vi "stupid put action.vi"(7 "transmit queue":refnum<queue>, 11 "application request in":T1) -> (0 "connection error":errorcluster)   [LabVIEW 2016]
uses:
  HTTP server/http request.ctl
  HTTP server/http method.ctl
  HTTP headers/http header data.ctl
  HTTP server/http response.ctl
  HTTP server/http response packet type.ctl
  HTTP headers/http add header to set.vi
  HTTP server/Basic HTTP server.lvclass
  HTTP headers/http headers.lvlib
  HTTP responder/http responder.lvclass
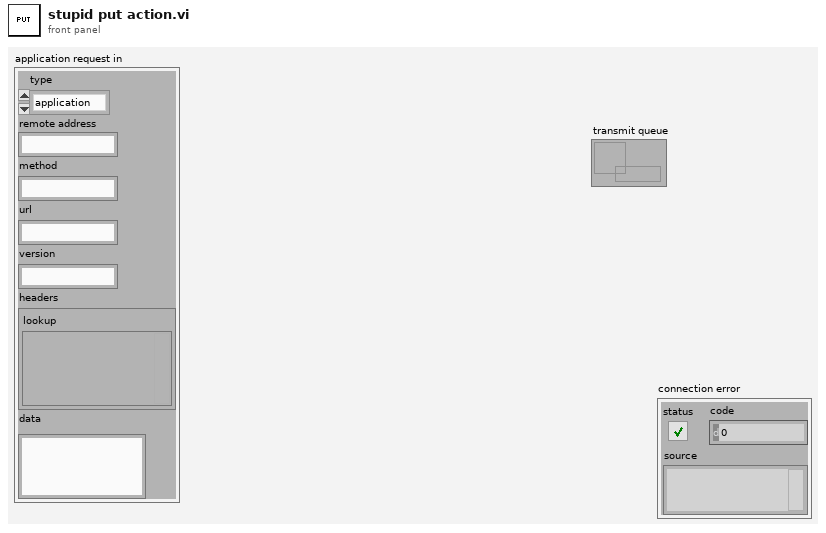
[diagram p1: front panel]
types:
  T1 = typedef "Basic HTTP server.lvclass/http request.ctl" = cluster{"type":T2, "remote address":string, "method":string, "url":string, "version":string, "headers":T3, "data":string}
  T2 = typedef "Basic HTTP server.lvclass/http method.ctl" = enum16{"application", "error", "upgrade", "expect"}
  T3 = typedef "http headers.lvlib/http header data.ctl" = cluster{"lookup":variant}
  T4 = typedef "Basic HTTP server.lvclass/http response packet type.ctl" = enum16{"full response", "header only", "data only", "last data", "raw output"}
  T5 = typedef "Basic HTTP server.lvclass/http response.ctl" = cluster{"packet type":T4, "reason code":u16, "status string":string, "headers":T3, "cookies":string[], "data":string}
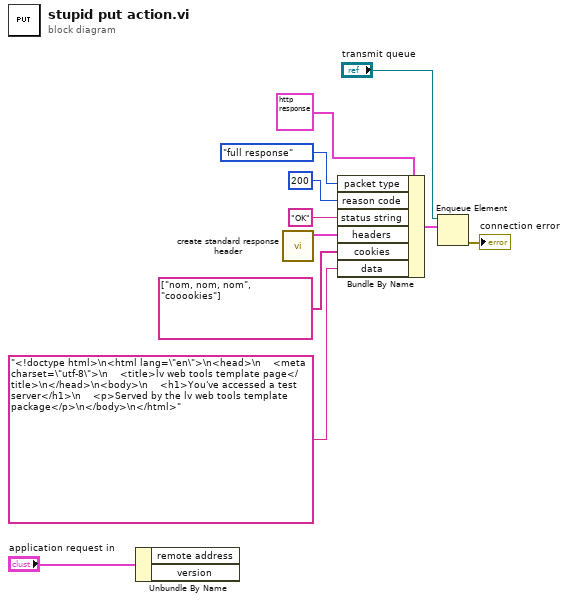
[diagram p0: block diagram]
diagram:
  n1 = Unbundle By Name("application request in") -> ()  [unwired: 2 out]
  n2 = call "create standard response header.vi"() -> ("default header"=w2:T3)  [unwired: 11 in]
  n3 = Bundle By Name(cluster=T5 {"packet type"=enum."full response", "reason code"=0, "status string"="", "headers"={"lookup"=variant}, "cookies"=[], "data"=""} ("application request"), "packet type"=http_response_packet_type."full response", "reason code"=u16 200, "status string"="OK", "headers"=w2, "cookies"=string[] ["nom, nom, nom", "cooookies"], "data"="<!doctype html>\n<html lang=\"en\">\n<head>\n    <meta charset=\"utf-8\">\n    <title>lv web tools template page</title>\n</head>\n<body>\n    <h1>You've accessed a test server</h1>\n    <p>Served by the lv web tools template package</p>\n</body>\n</html>") -> (w4:T5)
  n4 = Enqueue Element(queue="transmit queue", element=w4) -> (error out=→"connection error":errorcluster)  [unwired: 2 in, 2 out]
